vi "Coinc (SubVI).vi"(9 "paneCoord":cluster{"x start":i32, "y start":i32}, 10 "goalCoord":cluster{"x start":i32, "y start":i32}, 11 "startCoord":cluster{"x start":i32, "y start":i32}) -> (2 "goalCoinc":bool, 3 "startCoinc":bool)   [LabVIEW 2011]
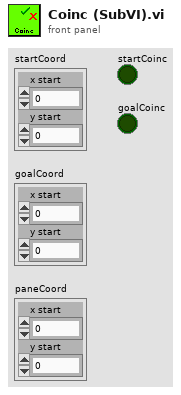
[diagram p1: front panel]
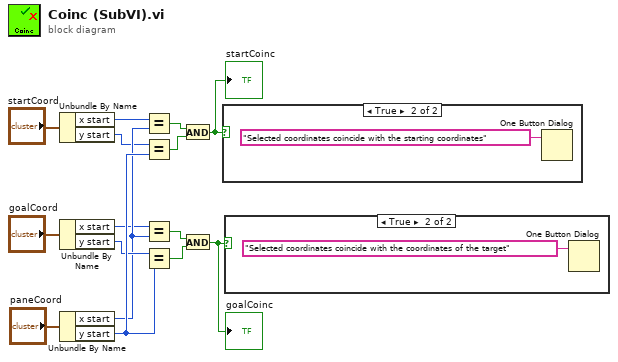
[diagram p0: block diagram]
diagram:
  n1 = Unbundle By Name("startCoord") -> ("x start"=w4:i32, "y start"=w5:i32)
  n2 = Unbundle By Name("goalCoord") -> ("x start"=w6:i32, "y start"=w8:i32)
  n3 = Unbundle By Name("paneCoord") -> ("x start"=w7:i32, "y start"=w9:i32)
  n4 = Equal?(x=w4, y=w7) -> (x = y?=w10:bool)
  n5 = Equal?(x=w5, y=w9) -> (x = y?=w11:bool)
  n6 = Equal?(x=w6, y=w7) -> (x = y?=w12:bool)
  n7 = Equal?(x=w8, y=w9) -> (x = y?=w13:bool)
  n8 = And(x=w10, y=w11) -> (x .and. y?=w14:bool)
  "startCoinc" <- w14
  n9 = And(x=w12, y=w13) -> (x .and. y?=w15:bool)
  "goalCoinc" <- w15
  n10 = case shown="True" w14 {
    frame False {
    }
    frame True {
      n11 = One Button Dialog(message="Selected coordinates coincide with the starting coordinates") -> ()  [unwired: 1 in, 1 out]
    }
  }
  n12 = case shown="True" w15 {
    frame False {
    }
    frame True {
      n13 = One Button Dialog(message="Selected coordinates coincide with the coordinates of the target") -> ()  [unwired: 1 in, 1 out]
    }
  }
